vi "sub_read_avi2.vi"(10 "Quality (750)":i32=750) -> (1 "frames":cluster{i32, "Data String":string}[](array[cluster]), 2 "Frames Per Second":u32)   [LabVIEW 2014]
panel:
  in  "Stop":bool
  out "Progress Bar":i32(slide) max=135 scale=1.0..135.0
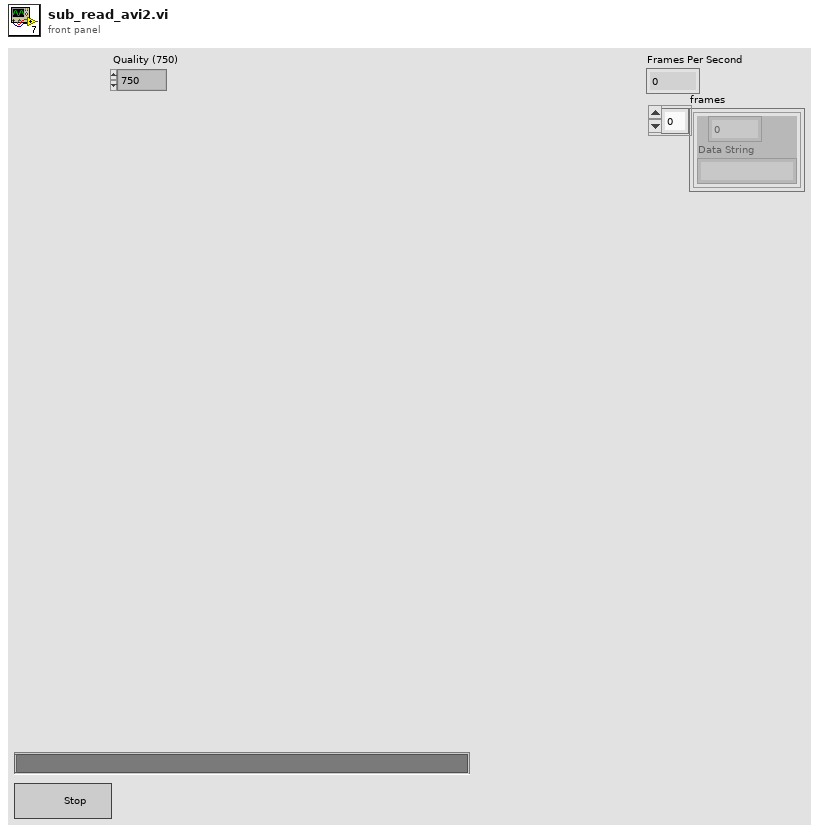
[diagram p1: front panel]
types:
  T1 = typedef "IMAQ AVI2 Refnum.ctl" = refnum<k20>
  T2 = typedef "Image Type" = u32
  T3 = cluster{"Width":u32, "Height":u32, "Frames Per Second":u32, "Codec":string, "Has Data":bool}
  T4 = typedef "IMAQ Image.ctl" = refnum<image>
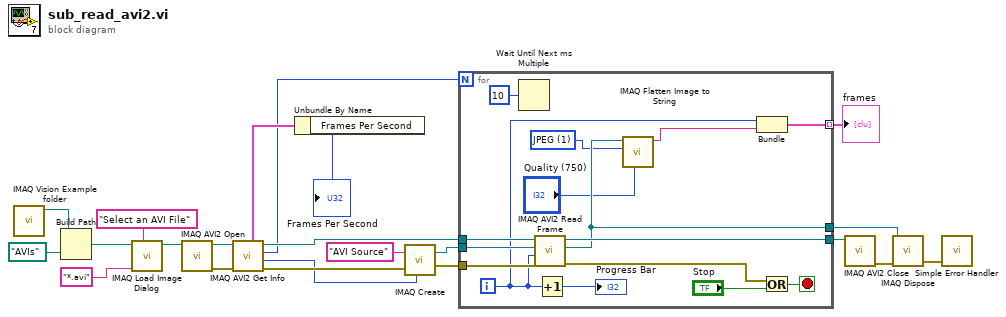
[diagram p0: block diagram]
diagram:
  n1 = call "IMAQ Vision Example folder.vi"() -> ("Example Image Path"=w9:path)  [unwired: 11 in]
  n2 = Build Path(base path=w9, name or relative path=path "AVIs") -> (appended path=w6:path)
  n3 = call "IMAQ Load Image Dialog"("Prompt"="Select an AVI File" ("prompt"), "Pattern"="*.avi", "Start Path"=w6) -> ("Path"=w5:path)  [unwired: 6 in, 2 out]
  n4 = call "IMAQ AVI2 Open"("AVI File Path"=w5) -> ("error out"=w19:errorcluster, "AVI Refnum"=w18:T1)  [unwired: 2 in, 7 out]
  n5 = call "IMAQ AVI2 Get Info"("error in (no error)"=w19, "AVI Refnum"=w18) -> ("error out"=w16:errorcluster, "Image Type"=w10:T2, "Number of Frames"=w3:u32, "AVI Refnum (duplicate)"=w13:T1, "Frame Data"=w20:T3)  [unwired: 5 out]
  n6 = Unbundle By Name(w20) -> ("Frames Per Second"=→"Frames Per Second":u32)
  n7 = call "IMAQ Create"("Image Name"="AVI Source", "Image Type"=w10, "error in (no error)"=w16) -> ("New Image"=w14:T4, "error out"=w15:errorcluster)  [unwired: 1 in, 1 out]
  n8 = for {
    N: w3 -> [_]
    tunnel: w14 -> [w36]
    tunnel: [w35] -> w17
    tunnel: w15 -> [w31]
    tunnel: w13 -> [w37]
    tunnel: [w27] -> w11
    tunnel: [w29] -> w1 mode=indexing
    i -> [w30]
    stop <- w33 stop-if-true
    w25 = 1 items=["None", "JPEG", "PACKED BINARY"] ("Compression (None)")
    n9 = Wait Until Next ms Multiple(millisecond multiple=u32 10) -> ()  [unwired: 1 out]
    n10 = call "IMAQ AVI2 Read Frame"("error in (no error)"=w31, "Frame Number"=w30, "Image"=w36, "AVI Refnum"=w37) -> ("error out"=w28:errorcluster, "Image Out"=w27:T4, "AVI Refnum (duplicate)"=w35:T1)  [unwired: 5 out]
    n11 = Increment(x=w30) -> (x+1=→"Progress Bar":i32)
    n12 = call "IMAQ Flatten Image to String"("Quality (750)"="Quality (750)", "Compression (None)"=w25, "Image"=w27) -> ("Data String"=w24:string)  [unwired: 7 in, 1 out]
    n13 = Bundle(w30, "Data String"=w24) -> (w29:cluster{i32, "Data String":string})  [unwired: 1 in]
    n14 = Or(x=w28, y="Stop") -> (x .or. y?=w33:bool)
  }
  "frames" <- w1
  n15 = call "IMAQ AVI2 Close"("AVI Refnum"=w17) -> ("error out"=w12:errorcluster)  [unwired: 1 in, 9 out]
  n16 = call "IMAQ Dispose"("Image"=w11, "error in (no error)"=w12) -> ("error out"=w21:errorcluster)  [unwired: 1 in, 3 out]
  n17 = call <vilib>:"Simple Error Handler.vi"("error in (no error)"=w21) -> ()  [unwired: 1 in, 8 out]
